vi "(Depricated) Publish Sample.vi"(8 "error in (no error)":errorcluster, 9 "Sample":refnum<class "Sample.lvclass">, 10 "Containers":T1[](array[typedef]), 11 "CO2 Actor in":refnum<class "CO2 Actor.lvclass">=refnum) -> (0 "error out":errorcluster, 3 "CO2 Actor in 2":refnum<class "CO2 Actor.lvclass">)   [LabVIEW 2015, in "CO2 Actor.lvclass"]
uses:
  CO2 Actor.lvclass
  subs/Sample/Sample.lvclass
  Controls/Sample Container.ctl
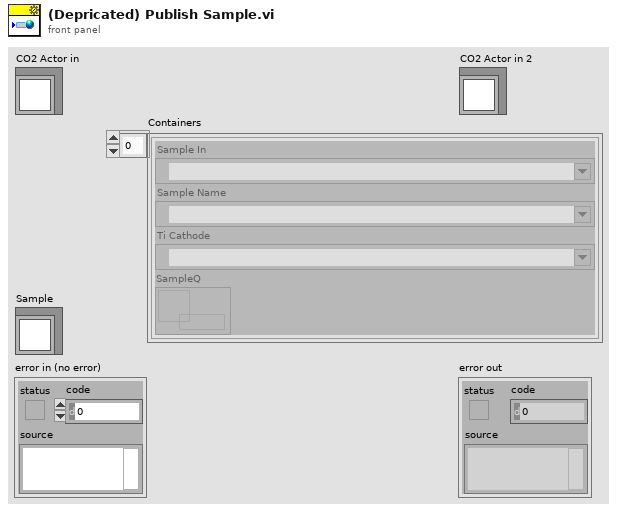
[diagram p1: front panel]
types:
  T1 = typedef "Sample Container.ctl" = cluster{"Sample In":refnum<k21>, "Sample Name":refnum<k21>, "Ti Cathode":refnum<k21>, "SampleQ":refnum<queue>}
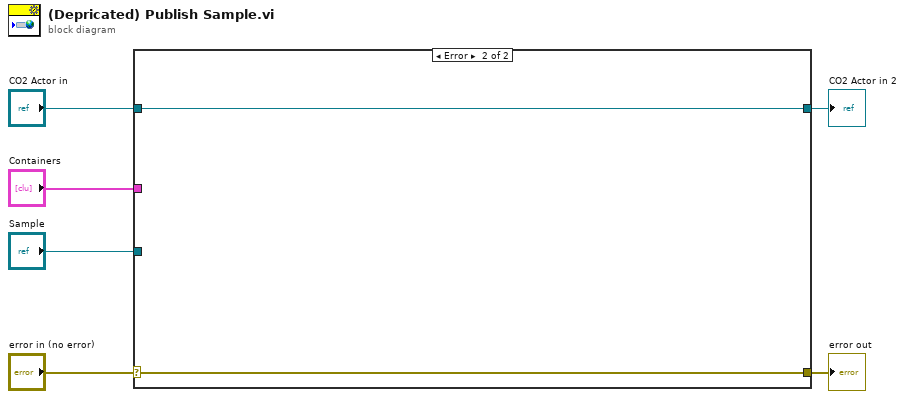
[diagram p0: block diagram]
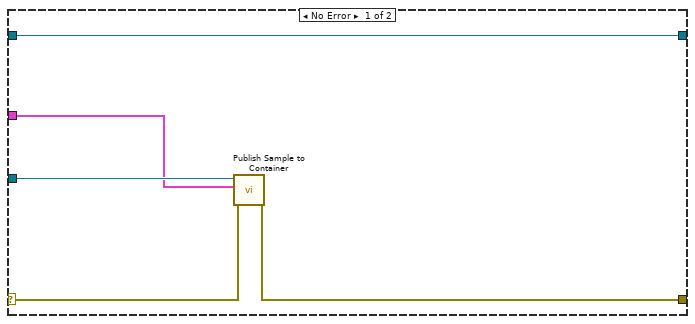
[diagram p2: hidden frame]
diagram:
  n1 = case shown="Error" "error in (no error)" {
    selector: "error in (no error)" -> [w9 w13]
    tunnel: [w8 w13] -> w5
    tunnel: [w11 w12] -> w3
    tunnel: "CO2 Actor in" -> [w11 w12]
    tunnel: "Containers" -> [w7 _]
    tunnel: "Sample" -> [w10 _]
    frame No Error {
      n2 = call "Publish Sample to Container.vi"("error in (no error)"=w9, "Containers"=w7, "Sample in"=w10) -> ("error out"=w8:errorcluster)  [unwired: 7 in, 1 out]
    }
    frame Error {
    }
  }
  "error out" <- w5
  "CO2 Actor in 2" <- w3
